vi "Set Button Mode.vi"(7 "Button Mode":i32, 8 "Explanation":refnum<vi>, 9 "Title":refnum<vi>, 10 "Glyph":refnum<vi>, 11 "Container Reference":refnum<vi>) -> ()   [LabVIEW 2021, in "myRIO Choice Button.xctl"]
uses:
  <vilib>/myRIO/Common/Instrument Driver Framework/Utilities/xctls/myRIO Choice Button/myRIO Choice Button.xctl
  <vilib>/Utility/miscctls.llb/LVPositionTypeDef.ctl
  <vilib>/Utility/miscctls.llb/LVBoundsTypeDef.ctl
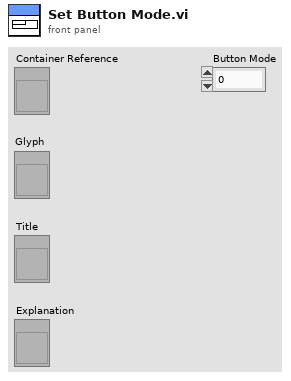
[diagram p1: front panel]
types:
  T1 = typedef "LVPositionTypeDef.ctl" = cluster{"Left":i32, "Top":i32}
  T2 = typedef "LVBoundsTypeDef.ctl" = cluster{"Width":u32, "Height":u32}
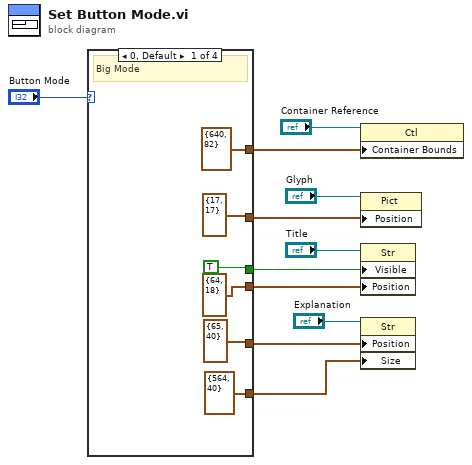
[diagram p0: block diagram]
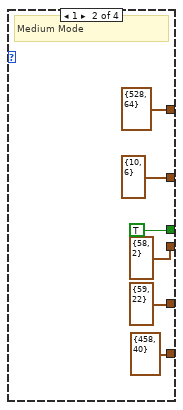
[diagram p2: hidden frame]
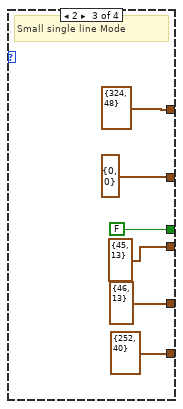
[diagram p3: hidden frame]
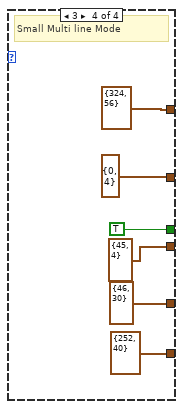
[diagram p4: hidden frame]
diagram:
  n1 = case shown="0, Default" "Button Mode" {
    tunnel: [TRUE ("Visible") TRUE ("Visible") FALSE ("Visible") TRUE ("Visible")] -> w4
    tunnel: [T1 {"Left"=17, "Top"=17} ("Position") T1 {"Left"=10, "Top"=6} ("Position") T1 {"Left"=0, "Top"=0} ("Position") T1 {"Left"=0, "Top"=4} ("Position")] -> w7
    tunnel: [T1 {"Left"=65, "Top"=40} ("Position") T1 {"Left"=59, "Top"=22} ("Position") T1 {"Left"=46, "Top"=13} ("Position") T1 {"Left"=46, "Top"=30} ("Position")] -> w9
    tunnel: [T2 {"Width"=564, "Height"=40} ("Size") T2 {"Width"=458, "Height"=40} ("Size") T2 {"Width"=252, "Height"=40} ("Size") T2 {"Width"=252, "Height"=40} ("Size")] -> w10
    tunnel: [T2 {"Width"=640, "Height"=82} ("XControl:Container Bounds") T2 {"Width"=528, "Height"=64} ("XControl:Container Bounds") T2 {"Width"=324, "Height"=48} ("XControl:Container Bounds") T2 {"Width"=324, "Height"=56} ("XControl:Container Bounds")] -> w11
    tunnel: [T1 {"Left"=64, "Top"=18} ("Position") T1 {"Left"=58, "Top"=2} ("Position") T1 {"Left"=45, "Top"=13} ("Position") T1 {"Left"=45, "Top"=4} ("Position")] -> w1
    frame 0, Default {
      # "Big Mode"
    }
    frame 1 {
      # "Medium Mode"
    }
    frame 2 {
      # "Small single line Mode"
    }
    frame 3 {
      # "Small Multi line Mode"
    }
  }
  n2 = property class="Ctl"(reference="Container Reference", "Container Bounds"=w11) -> ()  [unwired: 1 in, 2 out]
  n3 = property class="Pict"(reference="Glyph", "Position"=w7) -> ()  [unwired: 1 in, 2 out]
  n4 = property class="Str"(reference="Title", "Visible"=w4, "Position"=w1) -> ()  [unwired: 1 in, 2 out]
  n5 = property class="Str"(reference="Explanation", "Position"=w9, "Size"=w10) -> ()  [unwired: 1 in, 2 out]
